vi "Main-sequence.vi"(8 "error in":errorcluster) -> (0 "error out":errorcluster)   [LabVIEW 2019]
uses:
  _ctrl/create-rw-close.ctl
  _ctrl/rw.ctl
  _ctrl/init-w-close.ctl
  Durability/common/UI dev-operator.ctl
  _ctrl/init-r-stop.ctl
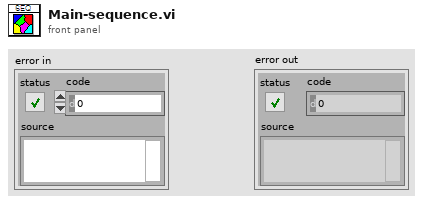
[diagram p1: front panel]
types:
  T1 = typedef "create-rw-close.ctl" = enum16{"create", "write", "read", "delete", "close"}
  T2 = typedef "init-w-close.ctl" = enum16{"open", "init", "write", "close"}
  T3 = typedef "rw.ctl" = enum16{"read", "write"}
  T4 = typedef "UI dev-operator.ctl" = enum16{"Testing", "Admin", "Operator", "Finish", "Ready"}
  T5 = typedef "init-r-stop.ctl" = enum16{"ini", "read", "stop"}
  T6 = typedef "sequence_single.ctl" = enum16{"Register", "RC", "B1", "B2", "B3", "Oper_LV", "Oper_HV", "ContR_LV"}
  T7 = typedef "Testing-info.ctl" = cluster{"전체채널수":u8, "현재채널번호":u8, "Irms":dbl, "입력전압":dbl, "입력전류":dbl, "출력전압":dbl, "출력전류":dbl, "온도":dbl, "제어단 단선":bool, "제어단 단락":bool, "제어단 특성변화":bool, "출력단 단선":bool, "출력단 단락":bool, "출력단 특성변화":bool, "출력단 전압":bool, "카운트 일치":bool, "Irms 판정":bool, "온도":bool, "테스트 회수":u32, "TestType":T6, "현재회수":u32, "Ch selection":cluster{"1ch":bool, "2ch":bool, "3ch":bool, "4ch":bool, "5ch":bool, "6ch":bool}, "반복":u32, "Path":path, "파일생성주기":u32, "start time":dbl, "stop time":dbl, "현재반복회수":u32, "NG":cluster{"입출력 카운트":bool, "출력전류RMS":bool}}
  T8 = cluster{"1ch":bool, "2ch":bool, "3ch":bool, "4ch":bool, "5ch":bool, "6ch":bool}
  T9 = typedef "ui_dev-operator.ctl" = cluster{"Operation stutus":refnum<vi>, "Test Status":refnum<vi>, "Setting":refnum<vi>, "Manual":refnum<vi>, "Main":refnum<vi>, "RCstart":refnum<vi>, "채널선택":refnum<vi>, "시험명":refnum<vi>, "Tab Control_manual":refnum<vi>, "시험 모드":refnum<vi>, "HW check":refnum<vi>, "login":refnum<vi>, "logout":refnum<vi>}
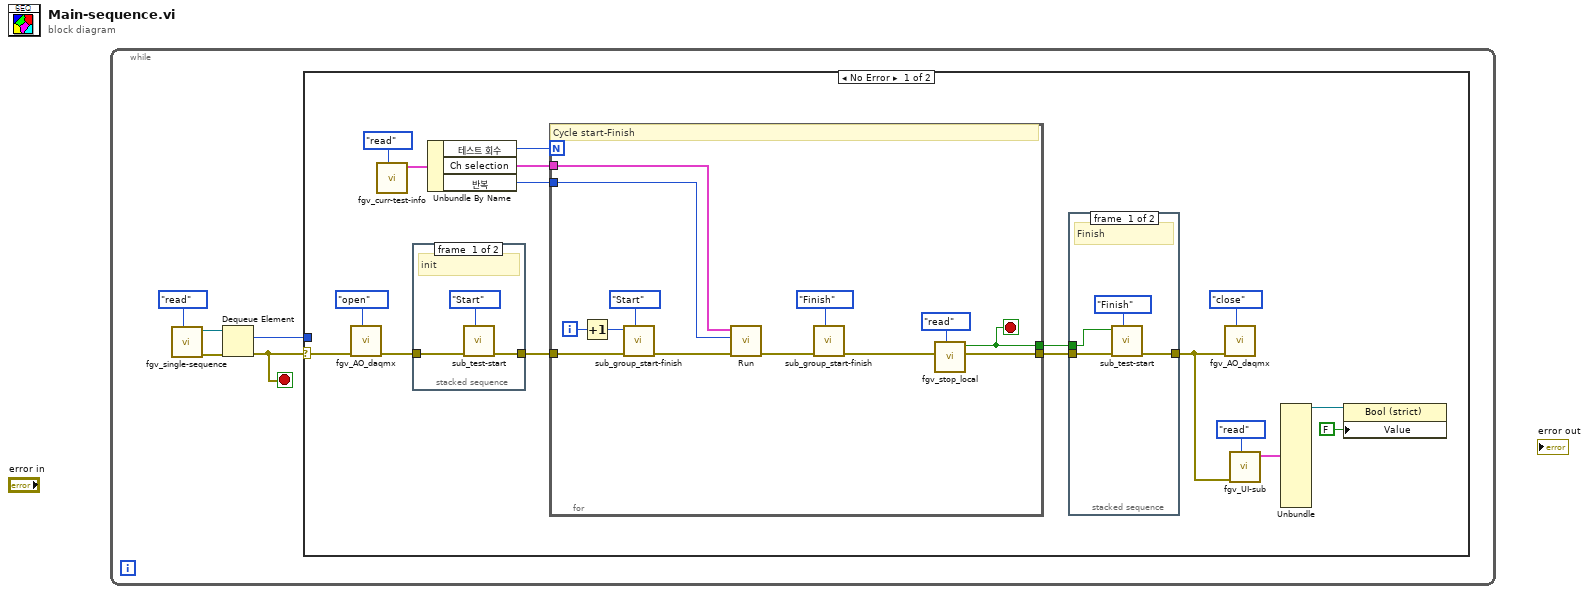
[diagram p0: block diagram]
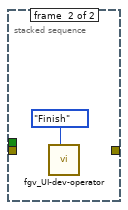
[diagram p2: hidden frame]
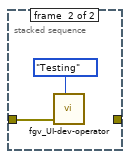
[diagram p3: hidden frame]
diagram:
  n1 = while {
    stop <- w2 stop-if-true
    n2 = call "fgv_single-sequence.vi"("cmd"=create-rw-close."read") -> ("error out"=w4:errorcluster, "queue out"=w3:refnum<queue>)  [unwired: 9 in]
    n3 = Dequeue Element(queue=w3, error in (no error)=w4) -> (element=w1:T6, error out=w2:errorcluster)  [unwired: 1 in, 2 out]
    n4 = case shown="No Error" w2 {
      selector: w2 -> [w8 _]
      tunnel: w1 -> [_ _]
      frame No Error {
        n5 = call "fgv_AO_daqmx.vi"("cmd"=init-w-close."open", "error in"=w8) -> ("error out"=w7:errorcluster)  [unwired: 9 in]
        n6 = call "fgv_curr-test-info.vi"("cmd"=rw."read") -> ("현재테스트 정보 2"=w18:T7)  [unwired: 10 in]
        n7 = stacked-sequence {
          tunnel: [w30 _] -> w13
          tunnel: w7 -> [w29 w31]
          frame #0 {
            # "init"
            n8 = call "sub_test-start.vi"("cmd"=enum16{"Start", "Finish"}."Start", "error in"=w29) -> ("error out"=w30:errorcluster)  [unwired: 9 in]
          }
          frame #1 {
            n9 = call "fgv_UI-dev-operator.vi"("cmd"=UI_dev-operator."Testing", "error in (no error)"=w31) -> ()  [unwired: 9 in, 1 out]
          }
        }
        n10 = Unbundle By Name(w18) -> ("테스트 회수"=w16:u32, "Ch selection"=w15:T8, "반복"=w10:u32)
        n11 = for {
          N: w16 -> [_]
          tunnel: [w35] -> w14
          tunnel: w15 -> [w43]
          tunnel: w13 -> [w39]
          tunnel: [w34] -> w11
          tunnel: w10 -> [w38]
          i -> [w45]
          stop <- w35 stop-if-true
          # "Cycle start-Finish"
          n12 = Increment(x=w45) -> (x+1=w44:i32)
          n13 = call "sub_group_start-finish.vi"("cmd"=enum16{"Start", "Finish"}."Start", "error in"=w39, "count"=w44) -> ("error out"=w33:errorcluster)  [unwired: 8 in]
          n14 = call "Run.vi"("error in (no error)"=w33, "반복"=w38, "Ch selection"=w43) -> ("error out"=w40:errorcluster)  [unwired: 7 in, 1 out]
          n15 = call "sub_group_start-finish.vi"("cmd"=enum16{"Start", "Finish"}."Finish", "error in"=w40) -> ("error out"=w36:errorcluster)  [unwired: 9 in]
          n16 = call "fgv_stop_local.vi"("cmd"=init-r-stop."read", "error in (no error)"=w36) -> ("error out"=w34:errorcluster, "stop"=w35:bool)  [unwired: 8 in]
        }
        n17 = stacked-sequence {
          tunnel: w14 -> [w23 _]
          tunnel: [w24 _] -> w12
          tunnel: w11 -> [w25 _]
          frame #0 {
            # "Finish"
            n18 = call "sub_test-start.vi"("cmd"=enum16{"Start", "Finish"}."Finish", "error in"=w25, "stop?"=w23) -> ("error out"=w24:errorcluster)  [unwired: 8 in]
          }
          frame #1 {
            n19 = call "fgv_UI-dev-operator.vi"("cmd"=UI_dev-operator."Finish") -> ()  [unwired: 10 in, 1 out]
          }
        }
        n20 = call "fgv_AO_daqmx.vi"("cmd"=init-w-close."close", "error in"=w12) -> ()  [unwired: 9 in, 1 out]
        n21 = call "fgv_UI-sub.vi"("cmd"=rw."read", "error in"=w12) -> ("output cluster 2"=w21:T9)  [unwired: 8 in, 1 out]
        n22 = Unbundle(w21) -> ("Operation stutus"=w22:refnum<vi>)  [unwired: 12 out]
        n23 = property class="Bool (strict)"(reference=w22, "Value"=FALSE) -> ()  [unwired: 1 in, 2 out]
      }
      frame Error {
      }
    }
  }
